vi "波形图与波形图表的比较及游标设置.vi"() -> ()   [LabVIEW 2010]
uses:
  <vilib>/Analysis/NI_AALBase.lvlib
panel:
  out "波形图":dbl[](graph) caption="Waveform Graph"
  out "Waveform Chart":dbl[](graph)
  # "(5)"
  # "(1)"
  # "(3)"
  # "(4)"
  # "(2)"
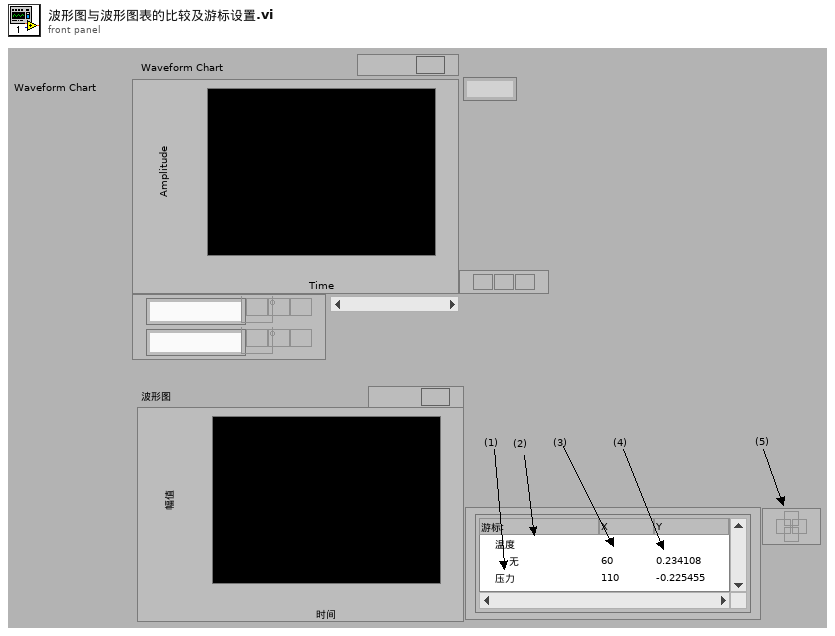
[diagram p1: front panel]
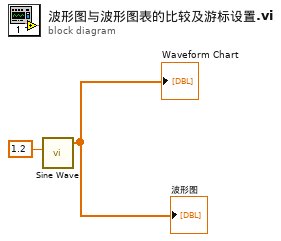
[diagram p0: block diagram]
diagram:
  n1 = call <vilib>:"Sine Wave.vi"("amplitude"=1.2) -> ("sine wave"=→"Waveform Chart" →"波形图":dbl[])  [unwired: 4 in, 2 out]
